vi "create.noManifest_endingTimestamp.vi"(9 "endingTimestamp":cluster{"seconds":i64, "nanos":i64, "picos":i64}, 10 "startingTimestamp":cluster{"seconds":i64, "nanos":i64, "picos":i64}) -> (3 "Timestamp Manifest":refnum<class "noManifest.lvclass">)   [LabVIEW 2020, in "nominal types.lvlib" / "timestampManifest.lvlib"]
uses:
  timestampManifest.lvlib
  noManifest/noManifest.lvclass
  endingTimestamp/endingTimestamp.lvclass
  C:/code/labview-client/lv_src/nominal types/timestampManifest/scaleParameter/scaleParameter.lvclass
  C:/code/labview-client/lv_src/Nominal Client/datasources/payload/payload.lvclass
  C:/code/labview-client/lv_src/nominal types/timestampManifest/endingTimestamp/endingTimestamp.lvclass
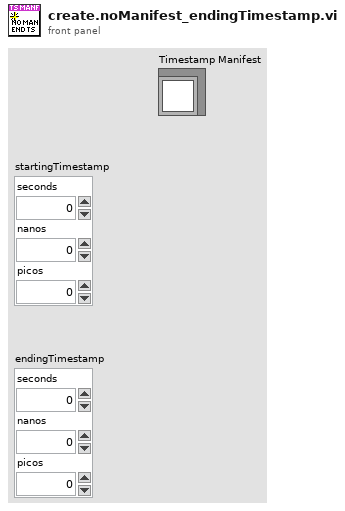
[diagram p1: front panel]
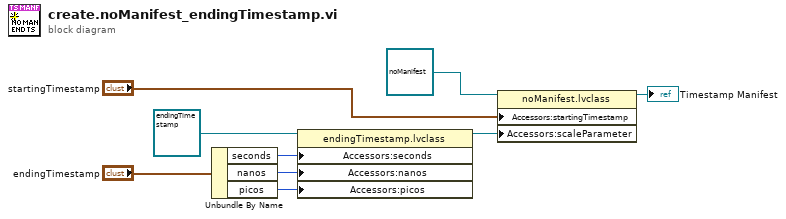
[diagram p0: block diagram]
diagram:
  n1 = Unbundle By Name("endingTimestamp") -> ("seconds"=w1:i64, "nanos"=w2:i64, "picos"=w3:i64)
  n2 = property class="endingTimestamp.lvclass"(reference=refnum<class "endingTimestamp.lvclass"> refnum ("nominal types.lvlib:timestampManifest.lvlib:endingTimestamp.lvclass"), "Accessors:seconds"=w1, "Accessors:nanos"=w2, "Accessors:picos"=w3) -> (reference out=w7:refnum<class "endingTimestamp.lvclass">)  [unwired: 1 in, 1 out]
  n3 = property class="noManifest.lvclass"(reference=refnum<class "noManifest.lvclass"> refnum ("nominal types.lvlib:timestampManifest.lvlib:noManifest.lvclass"), "Accessors:startingTimestamp"="startingTimestamp", "Accessors:scaleParameter"=w7) -> (reference out=→"Timestamp Manifest":refnum<class "noManifest.lvclass">)  [unwired: 1 in, 1 out]
